vi "Filter Spectra by Timestamps.vi"(8 "# Plots (10)":i32=10, 9 "Single Spectrum":cluster{"f0":dbl, "df":dbl, "magnitude":dbl[]}, 10 "Data Timestamp":dbl, 11 "Waterfall Age":dbl) -> (2 "Spectra to Plot":cluster{"f0":dbl, "df":dbl, "magnitude":dbl[]}[](array[cluster]), 3 "Spectra Plot with Timestamp":T1(array[cluster]))   [LabVIEW 2018, in "Fuel Farm.lvlib"]
uses:
  Fuel Farm.lvlib
  <vilib>/Analysis/baseanly.llb/Mean (DBL).vi
  <vilib>/Analysis/NI_AALBase.lvlib
panel:
  out "Waveform Graph 2":dbl[][](graph)
  in  "2D array":dbl[][](array[numeric])
  out "size(s) 2":i32[](array[numeric])
  out "size(s)":i32[](array[numeric])
  out "Waveform Graph":dbl[][](graph)
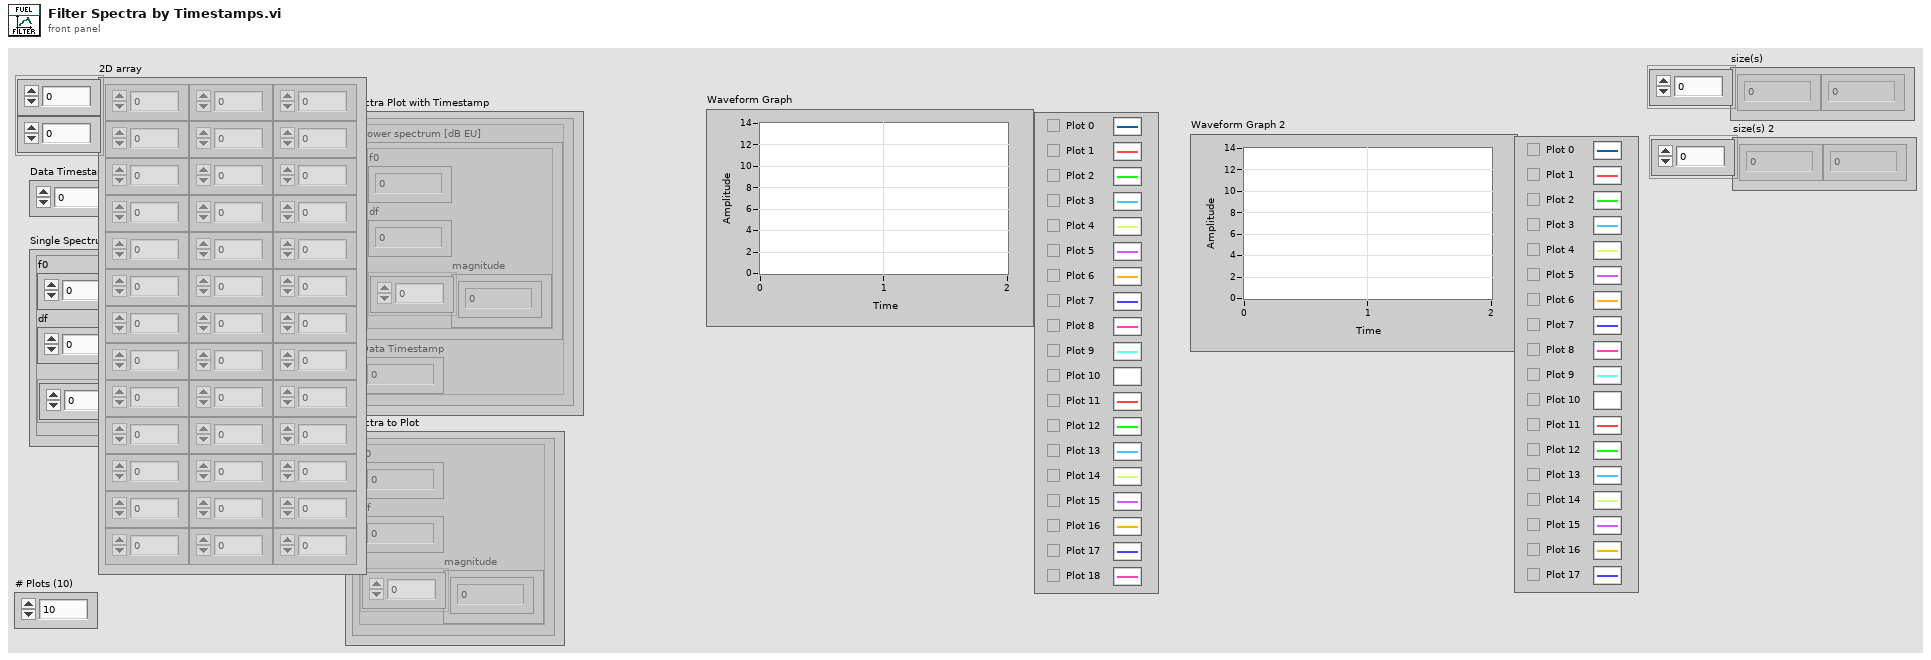
[diagram p1: front panel]
types:
  T1 = cluster{"power spectrum [dB EU]":cluster{"f0":dbl, "df":dbl, "magnitude":dbl[]}, "Data Timestamp":dbl}[]
  T2 = cluster{"power spectrum [dB EU]":cluster{"f0":dbl, "df":dbl, "magnitude":dbl[]}, "Data Tmstmp":dbl}
  T3 = cluster{"power spectrum [dB EU]":cluster{"f0":dbl, "df":dbl, "magnitude":dbl[]}, "Data Tmstmp":dbl}[]
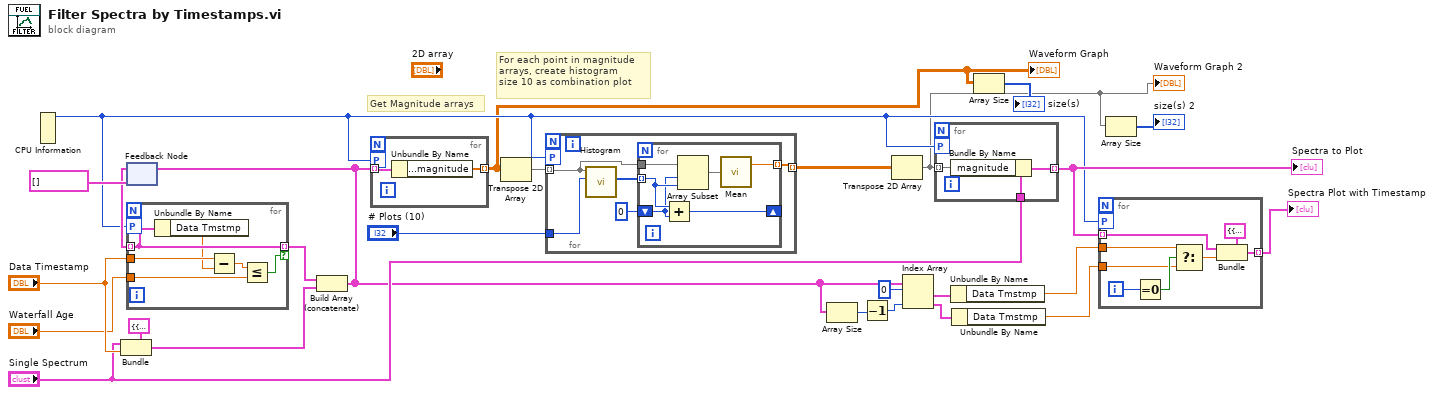
[diagram p0: block diagram]
diagram:
  # "For each point in magnitude\narrays, create histogram\nsize 10 as combination plot"
  # "Get Magnitude arrays"
  n1 = CPU Information() -> (4:w8:i32)  [unwired: 3 out]
  n2 = Bundle(cluster=T2 {"power spectrum [dB EU]"={"f0"=0.0, "df"=0.0, "magnitude"=[]}, "Data Tmstmp"=0.0}, "power spectrum [dB EU]"="Single Spectrum", "Data Tmstmp"="Data Timestamp") -> (w19:T2)
  n3 = feedback #1(T3 []) -> (w23:T3)
  n4 = for {
    tunnel: [w28] -> w22 mode=indexing if=w29
    tunnel: w23 -> [w28] mode=indexing
    tunnel: "Data Timestamp" -> [w32]
    tunnel: "Waterfall Age" -> [w30]
    workers-P: w8 -> [_]
    n5 = Unbundle By Name(w28) -> ("Data Tmstmp"=w27:dbl)
    n6 = Subtract(x=w32, y=w27) -> (x-y=w31:dbl)
    n7 = Less Or Equal?(x=w31, y=w30) -> (x <= y?=w29:bool)
  }
  n8 = Build Array (concatenate)(w22, w19) -> (w4:T3)
  n9 = feedback-in #1(w4) -> ()
  n10 = for {
    tunnel: w4 -> [w34] mode=indexing
    tunnel: [w33] -> w2 mode=indexing
    workers-P: w8 -> [_]
    n11 = Unbundle By Name(w34) -> ("power spectrum [dB EU].magnitude"=w33:dbl[])
  }
  "Waveform Graph" <- w2
  n12 = Transpose 2D Array(2D array=w2) -> (transposed array=w7:dbl[][])
  n13 = for {
    tunnel: w7 -> [w38] mode=indexing
    tunnel: [w36] -> w20 mode=indexing
    workers-P: w8 -> [_]
    tunnel: "# Plots (10)" -> [w35]
    n14 = call <vilib>:"Histogram.vi"("intervals"=w35, "X"=w38) -> ("Histogram: h(x)"=w39:i32[])  [unwired: 6 in, 3 out]
    n15 = for {
      tunnel: w39 -> [w43] mode=indexing
      tunnel: w38 -> [w45]
      shift-right: [w44] -> _
      shift-left: 0 -> [w42]
      tunnel: [w40] -> w36 mode=indexing
      n16 = Add(x=w43, y=w42) -> (x+y=w44:i32)
      n17 = Array Subset(array=w45, index=w42, length=w43) -> (w41:dbl[])
      n18 = call-poly <vilib>:"Mean.vi"("X"=w41) -> ("mean"=w40:dbl)  [unwired: 1 out]
    }
  }
  n19 = Array Size(array=w4) -> (size(s)=w18:i32)
  n20 = Decrement(x=w18) -> (x-1=w13:i32)
  n21 = Transpose 2D Array(2D array=w20) -> (transposed array=w3:dbl[][])
  "Waveform Graph 2" <- w3
  n22 = Index Array(array=w4, index #1=0 ("index"), index #2=w13) -> (element #1=w17:T2, element #2=w16:T2)
  n23 = for {
    workers-P: w8 -> [_]
    tunnel: w3 -> [w47] mode=indexing
    tunnel: "Single Spectrum" -> [w48]
    tunnel: [w46] -> w12 mode=indexing
    n24 = Bundle By Name(cluster=w48, "magnitude"=w47) -> (w46:cluster{"f0":dbl, "df":dbl, "magnitude":dbl[]})
  }
  "Spectra to Plot" <- w12
  n25 = Unbundle By Name(w17) -> ("Data Tmstmp"=w10:dbl)
  n26 = Unbundle By Name(w16) -> ("Data Tmstmp"=w9:dbl)
  n27 = Array Size(array=w2) -> (size(s)=→"size(s)":i32[])
  n28 = for {
    tunnel: w12 -> [w49] mode=indexing
    tunnel: [w52] -> w11 mode=indexing
    tunnel: w10 -> [w51]
    tunnel: w9 -> [w50]
    workers-P: w8 -> [_]
    i -> [w56]
    n29 = Equal To 0?(x=w56) -> (x = 0?=w55:bool)
    n30 = Select(t=w51, s=w55, f=w50) -> (s? t:f=w53:dbl)
    n31 = Bundle(cluster=T2 {"power spectrum [dB EU]"={"f0"=0.0, "df"=0.0, "magnitude"=[]}, "Data Tmstmp"=0.0}, "power spectrum [dB EU]"=w49, "Data Tmstmp"=w53) -> (w52:T2)
  }
  "Spectra Plot with Timestamp" <- w11
  n32 = Array Size(array=w3) -> (size(s)=→"size(s) 2":i32[])
